vi "rsscope_core_global.vi"() -> ()   [LabVIEW 2018] (continued)
 Only"=TRUE, "Identifier"="", "Descriptive Name"="Results", "Data Type"=0, "Command"="", "Access"=0, "Range Table"="", "Read Callback"="", "Write Callback"="", "Supported Models"="", "Instrument Options"="", "Flags"=0, "Help"="Queries selected result."}, {"Level"=4, "Class Only"=FALSE, "Identifier"="RSSCOPE_ATTR_TRIGGER_PMETER_MEASUREMENT_COMMON_RESULT", "Descriptive Name"="Trigger Common Measurement Result", "Data Type"=1, "Command"="TRPR:PMET:RES:COMM?", "Access"=0, "Range Table"="", "Read Callback"="", "Write Callback"="", "Supported Models"="", "Instrument Options"="", "Flags"=0, "Help"="Returns the common mode voltage - the mean voltage between the signal sockets and the ground socket.\n\nAvailable Repeated Capabilities:\nNone\n\nRemote-control command(s):\nTRPRobe:PMETer:RESults:COMMon?"}, {"Level"=4, "Class Only"=FALSE, "Identifier"="RSSCOPE_ATTR_TRIGGER_PMATER_MEASUREMENT_DIFFERENTIAL_RESULT", "Descriptive Name"="Trigger Differential Measurement Result", "Data Type"=1, "Command"="TRPR:PMET:RES:DIFF?", "Access"=0, "Range Table"="", "Read Callback"="", "Write Callback"="", "Supported Models"="", "Instrument Options"="", "Flags"=0, "Help"="Returns the differential voltage - the voltage between the positive and negative signal sockets.\n\nAvailable Repeated Capabilities:\nNone\n\nRemote-control command(s):\nTRPRobe:PMETer:RESults:DIFFerential?"}, {"Level"=4, "Class Only"=FALSE, "Identifier"="RSSCOPE_ATTR_TRIGGER_PMETER_MEASUREMENT_POSITIVE_RESULT", "Descriptive Name"="Trigger Single Ended Positive Measurement Result", "Data Type"=1, "Command"="TRPR:PMET:RES:POS?", "Access"=0, "Range Table"="", "Read Callback"="", "Write Callback"="", "Supported Models"="", "Instrument Options"="", "Flags"=0, "Help"="Returns the voltage that is measured between the negative signal socket and the ground.\n\nAvailable Repeated Capabilities:\nNone\n\nRemote-control command(s):\nTRPRobe:PMETer:RESults:POSitive?"}, {"Level"=4, "Class Only"=FALSE, "Identifier"="RSSCOPE_ATTR_TRIGGER_PMETER_MEASUREMENT_NEGATIVE_RESULT", "Descriptive Name"="Trigger Single Ended Negative Measurement Result", "Data Type"=1, "Command"="TRPR:PMET:RES:NEG?", "Access"=0, "Range Table"="", "Read Callback"="", "Write Callback"="", "Supported Models"="", "Instrument Options"="", "Flags"=0, "Help"="Returns the voltage that is measured between the negative signal socket and the ground.\n\nAvailable Repeated Capabilities:\nNone\n\nRemote-control command(s):\nTRPRobe:PMETer:RESults:NEGative?"}, {"Level"=4, "Class Only"=FALSE, "Identifier"="RSSCOPE_ATTR_TRIGGER_PMETER_MEASUREMENT_SINGLE_RESULT", "Descriptive Name"="Trigger Single Ended Measurement Result", "Data Type"=1, "Command"="TRPR:PMET:RES:SING?", "Access"=0, "Range Table"="", "Read Callback"="", "Write Callback"="", "Supported Models"="", "Instrument Options"="", "Flags"=0, "Help"="Returns the voltage measured between the probe tip and the ground.\n\nAvailable Repeated Capabilities:\nNone\n\nRemote-control command(s):\nTRPRobe:PMETer:RESults:SINGle?"}, {"Level"=1, "Class Only"=TRUE, "Identifier"="", "Descriptive Name"="Channel Subsystem", "Data Type"=0, "Command"="", "Access"=0, "Range Table"="", "Read Callback"="", "Write Callback"="", "Supported Models"="", "Instrument Options"="", "Flags"=0, "Help"="Channel-based attributes that you use to configure the channel subsystemof the oscilloscope.  All of the channel subsystem attributes are channel-based."}, {"Level"=2, "Class Only"=FALSE, "Identifier"="RSSCOPE_ATTR_CHANNEL_ENABLED", "Descriptive Name"="Channel Enabled", "Data Type"=3, "Command"="CHAN{Channel}:STAT", "Access"=2, "Range Table"="", "Read Callback"="", "Write Callback"="", "Supported Models"="", "Instrument Options"="", "Flags"=1, "Help"="Switches the channel signal on or off.\n\nAvailable Repeated Capabilities:\nChannel: CH1, CH2, CH3, CH4, CHExt\r\n\nRemote-control command(s):\nCHANnel<m>:STATe"}, {"Level"=2, "Class Only"=FALSE, "Identifier"="RSSCOPE_ATTR_VERTICAL_RANGE", "Descriptive Name"="Vertical Range", "Data Type"=1, "Command"="CHAN{Channel}:RANG", "Access"=2, "Range Table"="", "Read Callback"="", "Write Callback"="", "Supported Models"="", "Instrument Options"="", "Flags"=0, "Help"="Sets the voltage range across the 10 vertical divisions of the diagram.\n\nAvailable Repeated Capabilities:\nChannel: CH1, CH2, CH3, CH4, CHExt\r\n\nRemote-control command(s):\nCHANnel<m>:RANGe"}, {"Level"=2, "Class Only"=FALSE, "Identifier"="RSSCOPE_ATTR_VERTICAL_OFFSET", "Descriptive Name"="Vertical Offset", "Data Type"=1, "Command"="CHAN{Channel}:POS", "Access"=2, "Range Table"="rsscope_rngVerticalOffset", "Read Callback"="", "Write Callback"="", "Supported Models"="", "Instrument Options"="", "Flags"=0, "Help"="Sets the vertical position of the indicated channel and its horizontal axis in the window.\n\nAvailable Repeated Capabilities:\nChannel: CH1, CH2, CH3, CH4, CHExt\r\n\nRemote-control command(s):\nCHANnel<m>:POSition"}, {"Level"=2, "Class Only"=FALSE, "Identifier"="RSSCOPE_ATTR_CHANNEL_INVERT", "Descriptive Name"="Channel Invert", "Data Type"=3, "Command"="CHAN{Channel}:INV", "Access"=2, "Range Table"="", "Read Callback"="", "Write Callback"="", "Supported Models"="", "Instrument Options"="", "Flags"=0, "Help"="Turns the inversion of the signal amplitude on or off. To invert means to reflect the voltage values of all signal components against the ground level. If the inverted channel is the trigger source, the instrument triggers on the inverted signal.\n\nAvailable Repeated Capabilities:\nChannel: CH1, CH2, CH3, CH4, CHExt\r\n\nRemote-control command(s):\nCHANnel<m>:INVert"}, {"Level"=2, "Class Only"=FALSE, "Identifier"="RSSCOPE_ATTR_VERTICAL_COUPLING", "Descriptive Name"="Vertical Coupling", "Data Type"=0, "Command"="CHAN{Channel}:COUP", "Access"=2, "Range Table"="rsscope_rngVerticalCoupling", "Read Callback"="", "Write Callback"="", "Supported Models"="", "Instrument Options"="", "Flags"=0, "Help"="Selects the connection of the indicated channel signal.\n\nAvailable Repeated Capabilities:\nChannel: CH1, CH2, CH3, CH4, CHExt\r\n\nRemote-control command(s):\nCHANnel<m>:COUPling"}, {"Level"=2, "Class Only"=FALSE, "Identifier"="RSSCOPE_ATTR_VERTICAL_SCALE", "Descriptive Name"="Vertical Scale", "Data Type"=1, "Command"="CHAN{Channel}:SCAL", "Access"=2, "Range Table"="", "Read Callback"="", "Write Callback"="", "Supported Models"="", "Instrument Options"="", "Flags"=0, "Help"="Sets the vertical scale for the indicated channel.\n\nAvailable Repeated Capabilities:\nChannel: CH1, CH2, CH3, CH4, CHExt\r\n\nRemote-control command(s):\nCHANnel<m>:SCALe"}, {"Level"=2, "Class Only"=FALSE, "Identifier"="RSSCOPE_ATTR_CHANNEL_OFFSET", "Descriptive Name"="Channel Offset", "Data Type"=1, "Command"="CHAN{Channel}:OFFS", "Access"=2, "Range Table"="", "Read Callback"="", "Write Callback"="", "Supported Models"="", "Instrument Options"="", "Flags"=0, "Help"="The offset voltage is subtracted to correct an offset-affected signal.\n\nAvailable Repeated Capabilities:\nChannel: CH1, CH2, CH3, CH4, CHExt\r\n\nRemote-control command(s):\nCHANnel<m>:OFFSet"}, {"Level"=2, "Class Only"=FALSE, "Identifier"="RSSCOPE_ATTR_CHANNEL_BANDWIDTH_LIMIT", "Descriptive Name"="Channel Bandwidth Limit", "Data Type"=0, "Command"="CHAN{Channel}:BAND", "Access"=2, "Range Table"="rsscope_rngChannelBWLimit", "Read Callback"="", "Write Callback"="", "Supported Models"="", "Instrument Options"="", "Flags"=0, "Help"="Selects the bandwidth limit for the indicated channel.\n\nAvailable Repeated Capabilities:\nChannel: CH1, CH2, CH3, CH4, CHExt\r\n\nRemote-control command(s):\nCHANnel<m>:BANDwidth"}, {"Level"=2, "Class Only"=FALSE, "Identifier"="RSSCOPE_ATTR_CHANNEL_OVERLOAD", "Descriptive Name"="Channel Overload", "Data Type"=3, "Command"="CHAN{Channel}:OVER", "Access"=2, "Range Table"="", "Read Callback"="", "Write Callback"="", "Supported Models"="", "Instrument Options"="", "Flags"=0, "Help"="Retrieves the overload status of the specified channel from the status bit. When the overload problem is solved, the command resets the status bit. Use VI_FALSE to clear the overload condition.\n\nAvailable Repeated Capabilities:\nChannel: CH1, CH2, CH3, CH4, CHExt\r\n\nRemote-control command(s):\nCHANnel<m>:OVERload"}, {"Level"=2, "Class Only"=FALSE, "Identifier"="RSSCOPE_ATTR_CHANNEL_ANTIALIASING", "Descriptive Name"="Channel Antialiasing", "Data Type"=0, "Command"="CHAN{Channel}:AAFP", "Access"=2, "Range Table"="RsScope_rngAntialiasing", "Read Callback"="", "Write Callback"="", "Supported Models"="", "Instrument Options"="", "Flags"=0, "Help"="Activates the anti-aliasing filter. The filter removes spurious and undersampled components of the signal and thus provides additional bandwidth limitation. The command is available for R&S RTO2064 and models with bandwidth extension option B2xx. Filter setting is only possible in remote control.\n\nAvailable Repeated Capabilities:\nChannel: CH1, CH2, CH3, CH4, CHExt\r\n\nRemote-control command(s):\nCHANnel<m>:AAFPermanent"}, {"Level"=2, "Class Only"=FALSE, "Identifier"="RSSCOPE_ATTR_INPUT_IMPEDANCE", "Descriptive Name"="Input Impedance", "Data Type"=1, "Command"="CHAN{Channel}:IMP", "Access"=2, "Range Table"="rsscope_rngInputImpedance", "Read Callback"="", "Write Callback"="", "Supported Models"="", "Instrument Options"="", "Flags"=0, "Help"="Sets the impedance of the channel for power calculations and measurements.\n\nAvailable Repeated Capabilities:\nChannel: CH1, CH2, CH3, CH4, CHExt\r\n\nRemote-control command(s):\nCHANnel<m>:IMPedance"}, {"Level"=2, "Class Only"=FALSE, "Identifier"="RSSCOPE_ATTR_GROUND_CONNECTION_ENABLED", "Descriptive Name"="Ground Connection Enabled", "Data Type"=3, "Command"="CHAN{Channel}:GND", "Access"=2, "Range Table"="", "Read Callback"="", "Write Callback"="", "Supported Models"="", "Instrument Options"="", "Flags"=0, "Help"="Connects the signal to the ground.\n\nAvailable Repeated Capabilities:\nChannel: CH1, CH2, CH3, CH4, CHExt\r\n\nRemote-control command(s):\nCHANnel<m>:GND"}, {"Level"=2, "Class Only"=FALSE, "Identifier"="RSSCOPE_ATTR_DIGITAL_FILTER_STATE", "Descriptive Name"="Digital Filter State", "Data Type"=3, "Command"="CHAN{Channel}:DIGF:STAT", "Access"=2, "Range Table"="", "Read Callback"="", "Write Callback"="", "Supported Models"="", "Instrument Options"="", "Flags"=0, "Help"="Enables the DSP filter.\n\nAvailable Repeated Capabilities:\nChannel: CH1, CH2, CH3, CH4, CHExt\r\n\nRemote-control command(s):\nCHANnel<m>:DIGFilter:STATe"}, {"Level"=2, "Class Only"=FALSE, "Identifier"="RSSCOPE_ATTR_DIGITAL_FILTER_CUT_OFF", "Descriptive Name"="Digital Filter Cut Off", "Data Type"=1, "Command"="CHAN{Channel}:DIGF:CUT", "Access"=2, "Range Table"="rsscope_rngDSPCutOff", "Read Callback"="", "Write Callback"="", "Supported Models"="", "Instrument Options"="", "Flags"=0, "Help"="Sets the limit frequency of the Lowpass filter for input channels.\n\nAvailable Repeated Capabilities:\nChannel: CH1, CH2, CH3, CH4, CHExt\r\n\nRemote-control command(s):\nCHANnel<m>:DIGFilter:CUToff"}, {"Level"=2, "Class Only"=FALSE, "Identifier"="RSSCOPE_ATTR_EXTERNAL_ATTENUATION_SCALE", "Descriptive Name"="External Attenuation Scale", "Data Type"=0, "Command"="CHAN{Channel}:EATS", "Access"=2, "Range Table"="rsscope_rngEATScale", "Read Callback"="", "Write Callback"="", "Supported Models"="", "Instrument Options"="", "Flags"=0, "Help"="Selects the attenuation scale for an external divider.\n\nAvailable Repeated Capabilities:\nChannel: CH1, CH2, CH3, CH4, CHExt\r\n\nRemote-control command(s):\nCHANnel<m>:EATScale"}, {"Level"=2, "Class Only"=FALSE, "Identifier"="RSSCOPE_ATTR_EXTERNAL_ATTENUATION_VALUE", "Descriptive Name"="External Attenuation Value", "Data Type"=1, "Command"="CHAN{Channel}:EATT", "Access"=2, "Range Table"="", "Read Callback"="", "Write Callback"="", "Supported Models"="", "Instrument Options"="", "Flags"=0, "Help"="Sets the attenuation of an external voltage divider.\n\nAvailable Repeated Capabilities:\nChannel: CH1, CH2, CH3, CH4, CHExt\r\n\nRemote-control command(s):\nCHANnel<m>:EATTenuation"}, {"Level"=2, "Class Only"=TRUE, "Identifier"="", "Descriptive Name"="Waveform", "Data Type"=0, "Command"="", "Access"=0, "Range Table"="", "Read Callback"="", "Write Callback"="", "Supported Models"="", "Instrument Options"="", "Flags"=0, "Help"="Attributes that configure the waveform measurement."}, {"Level"=3, "Class Only"=FALSE, "Identifier"="RSSCOPE_ATTR_WAVEFORM_STATE", "Descriptive Name"="Waveform State", "Data Type"=3, "Command"="CHAN{Channel}:WAV{Waveform}", "Access"=2, "Range Table"="", "Read Callback"="", "Write Callback"="", "Supported Models"="", "Instrument Options"="", "Flags"=0, "Help"="Activates or deactivates a waveform.\n\nAvailable Repeated Capabilities:\nChannel: CH1, CH2, CH3, CH4, CHExt\r\nWaveform: W0, W1, W2, W3\r\n\nRemote-control command(s):\nCHANnel<m>[:WAVeform<n>][:STATe]"}, {"Level"=3, "Class Only"=FALSE, "Identifier"="RSSCOPE_ATTR_WAVEFORM_HEADER", "Descriptive Name"="Waveform Header", "Data Type"=2, "Command"="CHAN{Channel}:WAV{Waveform}:DATA:HEAD?", "Access"=0, "Range Table"="", "Read Callback"="", "Write Callback"="", "Supported Models"="", "Instrument Options"="", "Flags"=0, "Help"="Returns the header of channel waveform data. The header contains setup and acquisition settings.\n\nAvailable Repeated Capabilities:\nChannel: CH1, CH2, CH3, CH4, CHExt\r\nWaveform: W0, W1, W2, W3\r\n\nRemote-control command(s):\nCHANnel<m>[:WAVeform<n>]:DATA:HEADer?"}, {"Level"=3, "Class Only"=FALSE, "Identifier"="RSSCOPE_ATTR_ACQUISITION_TYPE", "Descriptive Name"="Acquisition Type", "Data Type"=0, "Command"="CHAN{Channel}:WAV{Waveform}:TYPE", "Access"=2, "Range Table"="rsscope_rngAcquisitionType", "Read Callback"="", "Write Callback"="", "Supported Models"="", "Instrument Options"="", "Flags"=0, "Help"="Selects the method to reduce the data stream of the ADC to a stream of waveform points with lower sample rate.\n\nAvailable Repeated Capabilities:\nChannel: CH1, CH2, CH3, CH4, CHExt\r\nWaveform: W0, W1, W2, W3\r\n\nRemote-control command(s):\nCHANnel<m>[:WAVeform<n>]:TYPE"}, {"Level"=3, "Class Only"=FALSE, "Identifier"="RSSCOPE_ATTR_WAVEFORM_ACQUISITION_TYPE", "Descriptive Name"="Waveform Acquisition Type", "Data Type"=0, "Command"="CHAN{Channel}:WAV{Waveform}:ARIT", "Access"=2, "Range Table"="rsscope_rngWaveformArithmetics", "Read Callback"="", "Write Callback"="", "Supported Models"="", "Instrument Options"="", "Flags"=0, "Help"="Selects the method to reduce the data stream of the ADC to a stream of waveform points with lower sample rate.\n\nAvailable Repeated Capabilities:\nChannel: CH1, CH2, CH3, CH4, CHExt\r\nWaveform: W0, W1, W2, W3\r\n\nRemote-control command(s):\nCHANnel<m>[:WAVeform<n>]:ARIThmetics"}, {"Level"=3, "Class Only"=FALSE, "Identifier"="RSSCOPE_ATTR_WAVEFORM_ACQUISITION_COUPLE_CHANNELS_ENABLED", "Descriptive Name"="Waveform Acquisition Couple Channels Enabled", "Data Type"=3, "Command"="ACQ:CDTA", "Access"=2, "Range Table"="", "Read Callback"="", "Write Callback"="", "Supported Models"="", "Instrument Options"="", "Flags"=0, "Help"="Sets the acquisition mode and the waveform arithmetic of all channels to the last set value. \nIf the acquisition settings are coupled, &apos;Multi waveform&apos; is not available, only one waveform per channel can be used.\n\nAvailable Repeated Capabilities:\nNone\n\nRemote-control command(s):\nACQuire:CDTA"}, {"Level"=3, "Class Only"=FALSE, "Identifier"="RSSCOPE_ATTR_MULTIWAVEFORM_ACQUISITION_ENABLED", "Descriptive Name"="Multiwaveform Acquisition Enabled", "Data Type"=3, "Command"="ACQ:MUW", "Access"=2, "Range Table"="", "Read Callback"="", "Write Callback"="", "Supported Models"="", "Instrument Options"="", "Flags"=0, "Help"="For each channel, up to three waveforms can be shown and analyzed. The decimation mode and the waveform arithmetic are specific for each waveform. So you can analyze several aspects of the signal: For example, waveform1 shows the peaks, and waveform2 shows the average of the signal.\n\nAvailable Repeated Capabilities:\nNone\n\nRemote-control command(s):\nACQuire:MUWaveform"}, {"Level"=2, "Class Only"=TRUE, "Identifier"="", "Descriptive Name"="Skew", "Data Type"=0, "Command"="", "Access"=0, "Range Table"="", "Read Callback"="", "Write Callback"="", "Supported Models"="", "Instrument Options"="", "Flags"=0, "Help"="Skew compensates signal propagation differences between channels caused by the different\nlength of cables, probes, and other sources. Correct skew values are important for\naccurate triggering and timing relations between channels."}, {"Level"=3, "Class Only"=FALSE, "Identifier"="RSSCOPE_ATTR_SKEW_OFFSET_STATE", "Descriptive Name"="Skew Offset State", "Data Type"=3, "Command"="CHAN{Channel}:SKEW:MAN", "Access"=2, "Range Table"="", "Read Callback"="", "Write Callback"="", "Supported Models"="", "Instrument Options"="", "Flags"=0, "Help"="If enabled, the &apos;Skew offset&apos; value is used for compensation. This improves horizontal and trigger accuracy.\n\nAvailable Repeated Capabilities:\nChannel: CH1, CH2, CH3, CH4, CHExt\r\n\nRemote-control command(s):\nCHANnel<m>:SKEW:MANual"}, {"Level"=3, "Class Only"=FALSE, "Identifier"="RSSCOPE_ATTR_SKEW_OFFSET", "Descriptive Name"="Skew Offset", "Data Type"=1, "Command"="CHAN{Channel}:SKEW:TIME", "Access"=2, "Range Table"="rsscope_rngSkewOffset", "Read Callback"="", "Write Callback"="", "Supported Models"="", "Instrument Options"="", "Flags"=0, "Help"="Sets an delay value, that is known from the circuit specifics but cannot be compensated by the instrument automatically. It affects only the selected input channel.\n\nAvailable Repeated Capabilities:\nChannel: CH1, CH2, CH3, CH4, CHExt\r\n\nRemote-control command(s):\nCHANnel<m>:SKEW:TIME"}, {"Level"=3, "Class Only"=FALSE, "Identifier"="RSSCOPE_ATTR_SKEW_EXTENSION_STATE", "Descriptive Name"="Skew Extension State", "Data Type"=3, "Command"="CHAN{Channel}:SKEW:EXT", "Access"=2, "Range Table"="", "Read Callback"="", "Write Callback"="", "Supported Models"="", "Instrument Options"="", "Flags"=0, "Help"="Enables a higher skew value range that can be set with RSSCOPE_ATTR_SKEW_OFFSET. The skew extension reduces the maximum number of acquisitions in the memory.\n\nAvailable Repeated Capabilities:\nChannel: CH1, CH2, CH3, CH4, CHExt\r\n\nRemote-control command(s):\nCHANnel<m>:SKEW:EXTended"}, {"Level"=3, "Class Only"=FALSE, "Identifier"="RSSCOPE_ATTR_PROBE_SKEW_STATE", "Descriptive Name"="Probe Skew State", "Data Type"=3, "Command"="PROB:SKES", "Access"=2, "Range Table"="", "Read Callback"="", "Write Callback"="", "Supported Models"="", "Instrument Options"="", "Flags"=0, "Help"="If enabled, the skew of all connected active probes is measured, displayed, and used for deskewing.\n\nAvailable Repeated Capabilities:\nNone\n\nRemote-control command(s):\nPROBe<m>:SKEState"}, {"Level"=2, "Class Only"=TRUE, "Identifier"="", "Descriptive Name"="Channel Coupling", "Data Type"=0, "Command"="", "Access"=0, "Range Table"="", "Read Callback"="", "Write Callback"="", "Supported Models"="", "Instrument Options"="", "Flags"=0, "Help"="This class contains methods for coupling the vertical settings of channels."}, {"Level"=3, "Class Only"=FALSE, "Identifier"="RSSCOPE_ATTR_COUPLE_VERTICAL_CHANNEL_SETTINGS_ENABLED", "Descriptive Name"="Couple Vertical Channel Settings Enabled", "Data Type"=3, "Command"="CHAN{Channel}:CPL C{CoupledChannel},", "Access"=1, "Range Table"="", "Read Callback"="", "Write Callback"="", "Supported Models"="", "Instrument Options"="", "Flags"=0, "Help"="Sets the vertical settings of the coupled channel to the values of the active channel.\n\nAvailable Repeated Capabilities:\nChannel: CH1, CH2, CH3, CH4, CHExt\r\nCoupledChannel: CplCH1, CplCH2, CplCH3, CplCH4\r\n\nRemote-control command(s):\nCHANnel<m>:CPLing"}, {"Level"=3, "Class Only"=FALSE, "Identifier"="RSSCOPE_ATTR_QUERY_VERTICAL_CHANNEL_SETTINGS_COUPLED", "Descriptive Name"="Query Vertical Channel Settings Coupled", "Data Type"=3, "Command"="CHAN{Channel}:CPL? C{CoupledChannel}", "Access"=0, "Range Table"="", "Read Callback"="", "Write Callback"="", "Supported Models"="", "Instrument Options"="", "Flags"=0, "Help"="Queries whether the vertical settings of the coupled channel are coupled to the values of the active channel.\n\nAvailable Repeated Capabilities:\nChannel: CH1, CH2, CH3, CH4, CHExt\r\nCoupledChannel: CplCH1, CplCH2, CplCH3, CplCH4\r\n\nRemote-control command(s):\nCHANnel<m>:CPLing?"}, {"Level"=2, "Class Only"=TRUE, "Identifier"="", "Descriptive Name"="Differential Signal", "Data Type"=0, "Command"="", "Access"=0, "Range Table"="", "Read Callback"="", "Write Callback"="", "Supported Models"="", "Instrument Options"="", "Flags"=0, "Help"="This class contains methods for configuration of differential signal channels."}, {"Level"=3, "Class Only"=FALSE, "Identifier"="RSSCOPE_ATTR_DIFFERENTIAL_SIGNAL_STATE", "Descriptive Name"="Differential Signal State", "Data Type"=3, "Command"="DIFF{DifferentialSignal}:STAT", "Access"=2, "Range Table"="", "Read Callback"="", "Write Callback"="", "Supported Models"="", "Instrument Options"="", "Flags"=0, "Help"="Activates the differential signal. Two differential signals are available.\n\nAvailable Repeated Capabilities:\nDifferentialSignal: Diff1, Diff2\r\n\nRemote-control command(s):\nDIFF<m>:STATe"}, {"Level"=3, "Class Only"=FALSE, "Identifier"="RSSCOPE_ATTR_DIFFERENTIAL_SIGNAL_POSITIVE_INPUT", "Descriptive Name"="Differential Signal Positive Input", "Data Type"=0, "Command"="DIFF{DifferentialSignal}:PSIG", "Access"=2, "Range Table"="RsScope_rngDifferentialInput", "Read Callback"="", "Write Callback"="", "Supported Models"="", "Instrument Options"="", "Flags"=0, "Help"="Select the analog input channel of the positive signal. For differential signal 1, analog Ch1 and Ch2 are used. Differential signal 2 uses Ch3 and Ch4.\n\nAvailable Repeated Capabilities:\nDifferentialSignal: Diff1, Diff2\r\n\nRemote-control command(s):\nDIFF<m>:PSIGnal"}, {"Level"=3, "Class Only"=FALSE, "Identifier"="RSSCOPE_ATTR_DIFFERENTIAL_SIGNAL_NEGATIVE_INPUT", "Descriptive Name"="Differential Signal Negative Input", "Data Type"=0, "Command"="DIFF{DifferentialSignal}:NSIG", "Access"=2, "Range Table"="RsScope_rngDifferentialInput", "Read Callback"="", "Write Callback"="", "Supported Models"="", "Instrument Options"="", "Flags"=0, "Help"="Select the analog input channel of the negative signal. For differential signal 1, analog Ch1 and Ch2 are used. Differential signal 2 uses Ch3 and Ch4.\n\nAvailable Repeated Capabilities:\nDifferentialSignal: Diff1, Diff2\r\n\nRemote-control command(s):\nDIFF<m>:NSIGnal"}, {"Level"=3, "Class Only"=FALSE, "Identifier"="RSSCOPE_ATTR_DIFFERENTIAL_SIGNAL_OUTPUT_A", "Descriptive Name"="Differential Signal Output A", "Data Type"=0, "Command"="DIFF{DifferentialSignal}:AOUT", "Access"=2, "Range Table"="RsScope_rngDifferentialOutput", "Read Callback"="", "Write Callback"="", "Supported Models"="", "Instrument Options"="", "Flags"=0, "Help"="Select the waveform that is the result of differential processing. 2 output waveforms per digital signal can be defined.\nThe number of output waveforms depends on deembedding.\n\nAvailable Repeated Capabilities:\nDifferentialSignal: Diff1, Diff2\r\n\nRemote-control command(s):\nDIFF<m>:AOUTput"}, {"Level"=3, "Class Only"=FALSE, "Identifier"="RSSCOPE_ATTR_DIFFERENTIAL_SIGNAL_OUTPUT_B", "Descriptive Name"="Differential Signal Output B", "Data Type"=0, "Command"="DIFF{DifferentialSignal}:BOUT", "Access"=2, "Range Table"="RsScope_rngDifferentialOutput", "Read Callback"="", "Write Callback"="", "Supported Models"="", "Instrument Options"="", "Flags"=0, "Help"="Select the waveform that is the result of differential processing. 2 output waveforms per digital signal can be defined.\nThe number of output waveforms depends on deembedding.\n\nAvailable Repeated Capabilities:\nDifferentialSignal: Diff1, Diff2\r\n\nRemote-control command(s):\nDIFF<m>:BOUTput"}, {"Level"=3, "Class Only"=FALSE, "Identifier"="RSSCOPE_ATTR_DIFFERENTIAL_COMMON_OFFSET", "Descriptive Name"="Differential Common Offset", "Data Type"=1, "Command"="DIFF{DifferentialSignal}:COMM:OFFS", "Access"=2, "Range Table"="RsScope_rngDifferentialCommonOffset", "Read Callback"="", "Write Callback"="", "Supported Models"="", "Instrument Options"="", "Flags"=0, "Help"="Set the offset of differential and common mode waveforms.\nVertical settings of P and N output are the vertical settings of the input channels.\n\nAvailable Repeated Capabilities:\nDifferentialSignal: Diff1, Diff2\r\n\nRemote-control command(s):\nDIFFerential<m>:COMMon:OFFSet"}, {"Level"=3, "Class Only"=FALSE, "Identifier"="RSSCOPE_ATTR_DIFFERENTIAL_OFFSET", "Descriptive Name"="Differential Offset", "Data Type"=1, "Command"="DIFF{DifferentialSignal}:DIFF:OFFS", "Access"=2, "Range Table"="RsScope_rngDifferentialCommonOffset", "Read Callback"="", "Write Callback"="", "Supported Models"="", "Instrument Options"="", "Flags"=0, "Help"="Set the offset of differential and common mode waveforms.\nVertical settings of P and N output are the vertical settings of the input channels.\n\nAvailable Repeated Capabilities:\nDifferentialSignal: Diff1, Diff2\r\n\nRemote-control command(s):\nDIFFerential<m>:DIFFerential:OFFSet"}, {"Level"=3, "Class Only"=FALSE, "Identifier"="RSSCOPE_ATTR_DIFFERENTIAL_COMMON_POSITION", "Descriptive Name"="Differential Common Position", "Data Type"=1, "Command"="DIFF{DifferentialSignal}:COMM:POS", "Access"=2, "Range Table"="RsScope_rngDifferentialPosition", "Read Callback"="", "Write Callback"="", "Supported Models"="", "Instrument Options"="", "Flags"=0, "Help"="Set the vertical position of differential and common mode waveforms.\nVertical settings of P and N output are the vertical settings of the input channels.\n\nAvailable Repeated Capabilities:\nDifferentialSignal: Diff1, Diff2\r\n\nRemote-control command(s):\nDIFFerential<m>:COMMon:POSition"}, {"Level"=3, "Class Only"=FALSE, "Identifier"="RSSCOPE_ATTR_DIFFERENTIAL_POSITION", "Descriptive Name"="Differential Position", "Data Type"=1, "Command"="DIFF{DifferentialSignal}:DIFF:POS", "Access"=2, "Range Table"="RsScope_rngDifferentialPosition", "Read Callback"="", "Write Callback"="", "Supported Models"="", "Instrument Options"="", "Flags"=0, "Help"="Set the vertical position of differential and common mode waveforms.\nVertical settings of P and N output are the vertical settings of the input channels.\n\nAvailable Repeated Capabilities:\nDifferentialSignal: Diff1, Diff2\r\n\nRemote-control command(s):\nDIFFerential<m>:DIFFerential:POSition"}, {"Level"=3, "Class Only"=FALSE, "Identifier"="RSSCOPE_ATTR_DIFFERENTIAL_COMMON_SCALE", "Descriptive Name"="Differential Common Scale", "Data Type"=1, "Command"="DIFF{DifferentialSignal}:COMM:SCAL", "Access"=2, "Range Table"="RsScope_rngDifferentialScale", "Read Callback"="", "Write Callback"="", "Supported Models"="", "Instrument Options"="", "Flags"=0, "Help"="Set the vertical scale of differential and common mode waveforms, respectively.\nVertical settings of P and N output are the vertical settings of the input channels.\n\nAvailable Repeated Capabilities:\nDifferentialSignal: Diff1, Diff2\r\n\nRemote-control command(s):\nDIFFerential<m>:COMMon:SCALe"}, {"Level"=3, "Class Only"=FALSE, "Identifier"="RSSCOPE_ATTR_DIFFERENTIAL_SCALE", "Descriptive Name"="Differential Scale", "Data Type"=1, "Command"="DIFF{DifferentialSignal}:DIFF:SCAL", "Access"=2, "Range Table"="RsScope_rngDifferentialScale", "Read Callback"="", "Write Callback"="", "Supported Models"="", "Instrument Options"="", "Flags"=0, "Help"="Set the vertical scale of differential and common mode waveforms, respectively.\nVertical settings of P and N output are the vertical settings of the input channels.\n\nAvailable Repeated Capabilities:\nDifferentialSignal: Diff1, Diff2\r\n\nRemote-control command(s):\nDIFFerential<m>:DIFFerential:SCALe"}, {"Level"=3, "Class Only"=FALSE, "Identifier"="RSSCOPE_ATTR_DIFFERENTIAL_COMMON_ENABLED", "Descriptive Name"="Differential Common Enabled", "Data Type"=3, "Command"="DIFF{DifferentialSignal}:COMM:STAT", "Access"=2, "Range Table"="", "Read Callback"="", "Write Callback"="", "Supported Models"="", "Instrument Options"="", "Flags"=0, "Help"="Enable the output waveforms if deembedding by software is active. In this case, all output waveforms can be displayed at the same time, and each output is enabled separately.\n\nAvailable Repeated Capabilities:\nDifferentialSignal: Diff1, Diff2\r\n\nRemote-control command(s):\nDIFFerential<m>:COMMon:STATe"}, {"Level"=3, "Class Only"=FALSE, "Identifier"="RSSCOPE_ATTR_DIFFERENTIAL_ENABLED", "Descriptive Name"="Differential Enabled", "Data Type"=3, "Command"="DIFF{DifferentialSignal}:DIFF:STAT", "Access"=2, "Range Table"="", "Read Callback"="", "Write Callback"="", "Supported Models"="", "Instrument Options"="", "Flags"=0, "Help"="Enable the output waveforms if deembedding by software is active. In this case, all output waveforms can be displayed at the same time, and each output is enabled separately.\n\nAvailable Repeated Capabilities:\nDifferentialSignal: Diff1, Diff2\r\n\nRemote-control command(s):\nDIFFerential<m>:DIFFerential:STATe"}, {"Level"=3, "Class Only"=FALSE, "Identifier"="RSSCOPE_ATTR_DIFFERENTIAL_NEGATIVE_SIGNAL_ENABLED", "Descriptive Name"="Differential Negative Signal Enabled", "Data Type"=3, "Command"="DIFF{DifferentialSignal}:NSIG:STAT", "Access"=2, "Range Table"="", "Read Callback"="", "Write Callback"="", "Supported Models"="", "Instrument Options"="", "Flags"=0, "Help"="Enable the output waveforms if deembedding by software is active. In this case, all output waveforms can be displayed at the same time, and each output is enabled separately.\n\nAvailable Repeated Capabilities:\nDifferentialSignal: Diff1, Diff2\r\n\nRemote-control command(s):\nDIFFerential<m>:NSIGnal:STATe"}, {"Level"=3, "Class Only"=FALSE, "Identifier"="RSSCOPE_ATTR_DIFFERENTIAL_POSITIVE_SIGNAL_ENABLED", "Descriptive Name"="Differential Positive Signal Enabled", "Data Type"=3, "Command"="DIFF{DifferentialSignal}:PSIG:STAT", "Access"=2, "Range Table"="", "Read Callback"="", "Write Callback"="", "Supported Models"="", "Instrument Options"="", "Flags"=0, "Help"="Enable the output waveforms if deembedding by software is active. In this case, all output waveforms can be displayed at the same time, and each output is enabled separately.\n\nAvailable Repeated Capabilities:\nDifferentialSignal: Diff1, Diff2\r\n\nRemote-control command(s):\nDIFFerential<m>:PSIGnal:STATe"}, {"Level"=3, "Class Only"=FALSE, "Identifier"="RSSCOPE_ATTR_DIFFERENTIAL_COUPLING_ENABLED", "Descriptive Name"="Differential Coupling Enabled", "Data Type"=3, "Command"="DIFF{DifferentialSignal}:COUP", "Access"=2, "Range Table"="", "Read Callback"="", "Write Callback"="", "Supported Models"="", "Instrument Options"="", "Flags"=0, "Help"="If enabled for a differential signal, the vertical scales of P, N, differential and common mode waveforms are coupled.\n\nAvailable Repeated Capabilities:\nDifferentialSignal: Diff1, Diff2\r\n\nRemote-control command(s):\nDIFFerential<m>:COUPling"}, {"Level"=1, "Class Only"=TRUE, "Identifier"="", "Descriptive Name"="High Definition", "Data Type"=0, "Command"="", "Access"=0, "Range Table"="", "Read Callback"="", "Write Callback"="", "Supported Models"="", "Instrument Options"="", "Flags"=0, "Help"="This class configures the high definition. Works only with option K-17."}, {"Level"=2, "Class Only"=FALSE, "Identifier"="RSSCOPE_ATTR_HIGH_DEFINITION_ENABLED", "Descriptive Name"="High Definition Enabled", "Data Type"=3, "Command"="HDEF:STAT", "Access"=2, "Range Table"="", "Read Callback"="", "Write Callback"="", "Supported Models"="", "Instrument Options"="", "Flags"=0, "Help"="Activates the high definition mode of the instrument.\n\nAvailable Repeated Capabilities:\nNone\n\nRemote-control command(s):\nHDEFinition:STATe"}, {"Level"=2, "Class Only"=FALSE, "Identifier"="RSSCOPE_ATTR_HIGH_DEFINITION_BANDWIDTH", "Descriptive Name"="High Definition Bandwidth", "Data Type"=1, "Command"="HDEF:BWID", "Access"=2, "Range Table"="RsScope_rngHighDefinitionBandwidth", "Read Callback"="", "Write Callback"="", "Supported Models"="", "Instrument Options"="", "Flags"=0, "Help"="Sets the filter bandwidth for the high definition mode.\n\nAvailable Repeated Capabilities:\nNone\n\nRemote-control command(s):\nHDEFinition:BWIDth"}, {"Level"=2, "Class Only"=FALSE, "Identifier"="RSSCOPE_ATTR_HIGH_DEFINITION_RESOLUTION", "Descriptive Name"="High Definition Resolution", "Data Type"=1, "Command"="HDEF:RES?", "Access"=0, "Range Table"="", "Read Callback"="", "Write Callback"="", "Supported Models"="", "Instrument Options"="", "Flags"=0, "Help"="Returns the resulting digital resolution in high definition mode.\n\nAvailable Repeated Capabilities:\nNone\n\nRemote-control command(s):\nHDEFinition:RESolution?"}, {"Level"=1, "Class Only"=TRUE, "Identifier"="", "Descriptive Name"="Triggering Subsystem", "Data Type"=0, "Command"="", "Access"=0, "Range Table"="", "Read Callback"="", "Write Callback"="", "Supported Models"="", "Instrument Options"="", "Flags"=0, "Help"="Attributes that control how the oscilloscope triggers."}, {"Level"=2, "Class Only"=FALSE, "Identifier"="RSSCOPE_ATTR_TRIGGER_TYPE", "Descriptive Name"="Trigger Type", "Data Type"=0, "Command"="TRIG{Trigger}:TYPE", "Access"=2, "Range Table"="rsscope_rngTriggerType", "Read Callback"="", "Write Callback"="", "Supported Models"="", "Instrument Options"="", "Flags"=0, "Help"="Sets the trigger type.\n\nAvailable Repeated Capabilities:\nTrigger: TrigA, TrigB, TrigR\r\n\nRemote-control command(s):\nTRIGger<m>:TYPE"}, {"Level"=2, "Class Only"=FALSE, "Identifier"="RSSCOPE_ATTR_TRIGGER_SOURCE", "Descriptive Name"="Trigger Source", "Data Type"=0, "Command"="TRIG{Trigger}:SOUR", "Access"=2, "Range Table"="rsscope_rngTriggerSource", "Read Callback"="", "Write Callback"="", "Supported Models"="", "Instrument Options"="", "Flags"=0, "Help"="Sets the trigger source for the selected trigger type.\n\nAvailable Repeated Capabilities:\nTrigger: TrigA, TrigB, TrigR\r\n\nRemote-control command(s):\nTRIGger<m>:SOURce[:SELect]"}, {"Level"=2, "Class Only"=FALSE, "Identifier"="RSSCOPE_ATTR_TRIGGER_SERIAL_BUS_SOURCE", "Descriptive Name"="Trigger Serial Bus Source", "Data Type"=0, "Command"="TRIG{Trigger}:SOUR:SBS", "Access"=2, "Range Table"="RsScope_rngTriggerSerialBus", "Read Callback"="", "Write Callback"="", "Supported Models"="", "Instrument Options"="", "Flags"=0, "Help"="Selects the serial bus to be triggered on.\n\nAvailable Repeated Capabilities:\nTrigger: TrigA, TrigB, TrigR\r\n\nRemote-control command(s):\nTRIGger<m>:SOURce:SBSelect"}, {"Level"=2, "Class Only"=FALSE, "Identifier"="RSSCOPE_ATTR_TRIGGER_MODIFIER", "Descriptive Name"="Trigger Modifier", "Data Type"=0, "Command"="TRIG{Trigger}:MODE", "Access"=2, "Range Table"="rsscope_rngTriggerMode", "Read Callback"="", "Write Callback"="", "Supported Models"="", "Instrument Options"="", "Flags"=0, "Help"="Sets the trigger mode. The trigger mode determines the behaviour of the instrument if no trigger occurs.\n\nAvailable Repeated Capabilities:\nTrigger: TrigA, TrigB, TrigR\r\n\nRemote-control command(s):\nTRIGger<m>:MODE"}, {"Level"=2, "Class Only"=FALSE, "Identifier"="RSSCOPE_ATTR_TRIGGER_LEVEL_AUTO_FIND", "Descriptive Name"="Trigger Level Auto Find", "Data Type"=4, "Command"="TRIG{Trigger}:FIND", "Access"=1, "Range Table"="", "Read Callback"="", "Write Callback"="", "Supported Models"="", "Instrument Options"="", "Flags"=0, "Help"="Sets the trigger level automatically. The attribute is not available for an external trigger source.\n\nAvailable Repeated Capabilities:\nTrigger: TrigA, TrigB, TrigR\r\n\nRemote-control command(s):\nTRIGger<m>:FINDlevel"}, {"Level"=2, "Class Only"=FALSE, "Identifier"="RSSCOPE_ATTR_TRIGGER_EVENT_COUPLING", "Descriptive Name"="Trigger Event Coupling", "Data Type"=3, "Command"="TRIG{Trigger}:ECO", "Access"=2, "Range Table"="", "Read Callback"="", "Write Callback"="", "Supported Models"="", "Instrument Options"="", "Flags"=0, "Help"="Sets the trigger levels of the channels to the values of the indicated event.\n\nAvailable Repeated Capabilities:\nTrigger: TrigA, TrigB, TrigR\r\n\nRemote-control command(s):\nTRIGger<m>:ECOupling"}, {"Level"=2, "Class Only"=FALSE, "Identifier"="RSSCOPE_ATTR_TRIGGER_SOURCE_COUPLING", "Descriptive Name"="Trigger Source Coupling", "Data Type"=3, "Command"="TRIG{Trigger}:SCO", "Access"=2, "Range Table"="", "Read Callback"="", "Write Callback"="", "Supported Models"="", "Instrument Options"="", "Flags"=0, "Help"="Sets the trigger levels of all channels to the value of channel 1 for the indicated trigger event. Only applies to the A-trigger.\n\nAvailable Repeated Capabilities:\nTrigger: TrigA, TrigB, TrigR\r\n\nRemote-control command(s):\nTRIGger<m>:SCOupling"}, {"Level"=2, "Class Only"=FALSE, "Identifier"="RSSCOPE_ATTR_TRIGGER_LINES_DISPLAY", "Descriptive Name"="Trigger Lines Display", "Data Type"=3, "Command"="DISP:TRIG:LIN", "Access"=2, "Range Table"="", "Read Callback"="", "Write Callback"="", "Supported Models"="", "Instrument Options"="", "Flags"=0, "Help"="Hides or shows the trigger levels in the diagrams.\n\nAvailable Repeated Capabilities:\nNone\n\nRemote-control command(s):\nDISPlay:TRIGger:LINes"}, {"Level"=2, "Class Only"=FALSE, "Identifier"="RSSCOPE_ATTR_TRIGGER_OUT_STATE", "Descriptive Name"="Trigger Out State", "Data Type"=3, "Command"="TRIG:OUT:STAT", "Access"=2, "Range Table"="", "Read Callback"="", "Write Callback"="", "Supported Models"="", "Instrument Options"="", "Flags"=0, "Help"="Enables/disbales the trigger out signal that is provided to the EXT TRIGGER OUT connector on the rear panel when a trigger occurs.\n\nAvailable Repeated Capabilities:\nNone\n\nRemote-control command(s):\nTRIGger<m>:OUT:STATe"}, {"Level"=2, "Class Only"=FALSE, "Identifier"="RSSCOPE_ATTR_TRIGGER_OUT_ACTION", "Descriptive Name"="Trigger Out Action", "Data Type"=0, "Command"="TRIG{Trigger}:OUT:ACT", "Access"=2, "Range Table"="RsScope_rngTriggerOutAction", "Read Callback"="", "Write Callback"="", "Supported Models"="", "Instrument Options"="", "Flags"=0, "Help"="Enables/disbales the trigger out signal that is provided to the [Trigger Out] connector on the rear panel when a trigger occurs.\n\nAvailable Repeated Capabilities:\nTrigger: TrigA, TrigB, TrigR\r\n\nRemote-control command(s):\nTRIGger<m>:OUT:ACTion"}, {"Level"=2, "Class Only"=FALSE, "Identifier"="RSSCOPE_ATTR_TRIGGER_OUT_POLARITY", "Descriptive Name"="Trigger Out Polarity", "Data Type"=0, "Command"="TRIG:OUT:POL", "Access"=2, "Range Table"="rsscope_rngPolarity", "Read Callback"="", "Write Callback"="", "Supported Models"="", "Instrument Options"="", "Flags"=0, "Help"="Sets the polarity of the trigger out pulse.\n\nAvailable Repeated Capabilities:\nNone\n\nRemote-control command(s):\nTRIGger<m>:OUT:POLarity"}, {"Level"=2, "Class Only"=FALSE, "Identifier"="RSSCOPE_ATTR_TRIGGER_OUT_PULSE_LENGTH", "Descriptive Name"="Trigger Out Pulse Length", "Data Type"=1, "Command"="TRIG:OUT:PLEN", "Access"=2, "Range Table"="rsscope_rngTriggerOutPulseLength", "Read Callback"="", "Write Callback"="", "Supported Models"="", "Instrument Options"="", "Flags"=0, "Help"="Sets the length of the trigger out pulse.\n\nAvailable Repeated Capabilities:\nNone\n\nRemote-control command(s):\nTRIGger<m>:OUT:PLENgth"}, {"Level"=2, "Class Only"=FALSE, "Identifier"="RSSCOPE_ATTR_TRIGGER_OUT_DELAY", "Descriptive Name"="Trigger Out Delay", "Data Type"=1, "Command"="TRIG:OUT:DEL", "Access"=2, "Range Table"="", "Read Callback"="", "Write Callback"="", "Supported Models"="", "Instrument Options"="", "Flags"=0, "Help"="Sets the delay of the first pulse edge to the trigger point. The setting is not available if a mask test or measurement is running and the on-violation event is set to trigger out pulse.\n\nAvailable Repeated Capabilities:\nNone\n\nRemote-control command(s):\nTRIGger<m>:OUT:DELay"}, {"Level"=2, "Class Only"=FALSE, "Identifier"="RSSCOPE_ATTR_TRIGGER_EVENT_BEEP", 
